vi "pDataBuffer.vi"() -> ()   [LabVIEW 2020]
panel:
  in  "pDataBuffer":u16[](array[numeric])=array[32768 elements]
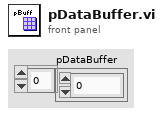
[diagram p1: front panel]
diagram:
